vi "absolute_relative.vi"() -> ()   [LabVIEW 2017]
uses:
  <vilib>/Utility/file.llb/Read Delimited Spreadsheet (string).vi
  <vilib>/Utility/file.llb/Write Delimited Spreadsheet (string).vi
panel:
  in  "Remove_dataset":path
  in  "Absolute_dataset":path
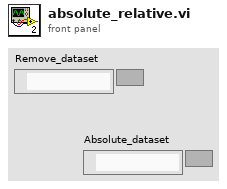
[diagram p1: front panel]
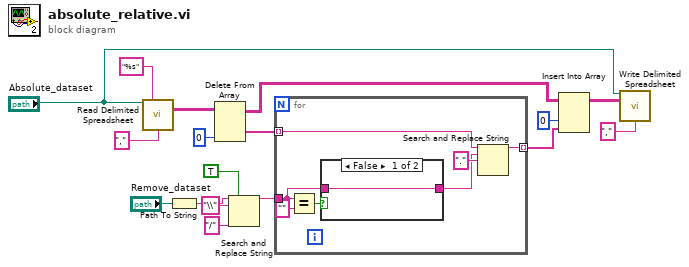
[diagram p0: block diagram]
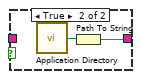
[diagram p2: hidden frame]
diagram:
  n1 = call-poly <vilib>:"Read Delimited Spreadsheet.vi"("file path (dialog if empty)"="Absolute_dataset", "format (%s)"="%s" ("format (%.3f)"), "delimiter (\\t)"="," ("delimiter (\\t)")) -> ("all rows"=w15:string[][])  [unwired: 7 in, 5 out]
  n2 = Path To String(path="Remove_dataset") -> (string=w11:string)
  n3 = Delete From Array(array=w15, index (col)=0 ("disabled index (col)")) -> (deleted portion=w14:string[], array with subset deleted=w6:string[][])  [unwired: 2 in]
  n4 = Search and Replace String(replace all?=TRUE ("replace all? (F)"), input string=w11, search string="\\", replace string="/" ("replace string (\"\")")) -> (result string=w12:string)  [unwired: 4 in, 3 out]
  n5 = for {
    tunnel: w14 -> [w23] mode=indexing
    tunnel: [w22] -> w5 mode=indexing
    tunnel: w12 -> [w19]
    n6 = Equal?(x=w19, y="") -> (x = y?=w21:bool)
    n7 = case shown="False" w21 {
      tunnel: [w25 w26] -> w18
      tunnel: w19 -> [w25 _]
      frame False {
      }
      frame True {
        n8 = call <vilib>:"Application Directory.vi"() -> ("Application Directory"=w27:path)
        n9 = Path To String(path=w27) -> (string=w26:string)
      }
    }
    n10 = Search and Replace String(input string=w23, search string=w18, replace string="." ("replace string (\"\")")) -> (result string=w22:string)  [unwired: 5 in, 3 out]
  }
  n11 = Insert Into Array(array=w6, index (col)=0 ("disabled index (col)"), new element=w5) -> (w3:string[][])  [unwired: 1 in]
  n12 = call-poly <vilib>:"Write Delimited Spreadsheet.vi"("file path (dialog if empty)"="Absolute_dataset", "2D data"=w3, "delimiter (\\t)"="," ("delimiter (\\t)")) -> ()  [unwired: 11 in, 2 out]
